vi "BMU诊断标定.vi"(8 "CAN端口":u16(ring), 9 "设备索引号":u16(ring), 10 "CAN卡类型":u32(ring)=21) -> ()   [LabVIEW 2013] (continued)
                              n3531 = control-ref of="项目信息"() -> (w5062:refnum<vi>)
                              n3532 = for {
                                N: w5055 -> [_]
                                tunnel: [""] -> w5061 mode=indexing
                              }
                              n3533 = Multiply(x=u8 1, y=w5056) -> (x*y=w5058:dbl)
                              n3534 = Add(x=w5058, y=u8 21) -> (x+y=w5054:dbl)
                              n3535 = call "表格数据输入-8.6.vi"("行数"=w5054, "列数"=u32 1, "字符串数组"=w5061, "表格引用"=w5062) -> ()  [unwired: 8 in]
                            }
                            frame "温度个数" {
                              n3536 = local read "从板个数"() -> (w5066:dbl)
                              n3537 = Increment(x=w5066) -> (x+1=w5065:dbl)
                              n3538 = control-ref of="项目信息"() -> (w5072:refnum<vi>)
                              n3539 = for {
                                N: w5065 -> [_]
                                tunnel: [""] -> w5071 mode=indexing
                              }
                              n3540 = Multiply(x=u8 2, y=w5066) -> (x*y=w5068:dbl)
                              n3541 = Add(x=w5068, y=u8 22) -> (x+y=w5064:dbl)
                              n3542 = call "表格数据输入-8.6.vi"("行数"=w5064, "列数"=u32 1, "字符串数组"=w5071, "表格引用"=w5072) -> ()  [unwired: 8 in]
                            }
                            frame "温度起始值" {
                              n3543 = local read "从板个数"() -> (w5076:dbl)
                              n3544 = Increment(x=w5076) -> (x+1=w5075:dbl)
                              n3545 = control-ref of="项目信息"() -> (w5082:refnum<vi>)
                              n3546 = for {
                                N: w5075 -> [_]
                                tunnel: [""] -> w5081 mode=indexing
                              }
                              n3547 = Multiply(x=u8 3, y=w5076) -> (x*y=w5078:dbl)
                              n3548 = Add(x=w5078, y=u8 23) -> (x+y=w5074:dbl)
                              n3549 = call "表格数据输入-8.6.vi"("行数"=w5074, "列数"=u32 1, "字符串数组"=w5081, "表格引用"=w5082) -> ()  [unwired: 8 in]
                            }
                            frame "保险位置" {
                              n3550 = local read "从板个数"() -> (w5086:dbl)
                              n3551 = control-ref of="项目信息"() -> (w5092:refnum<vi>)
                              n3552 = for {
                                N: 10 -> [_]
                                tunnel: [""] -> w5091 mode=indexing
                              }
                              n3553 = Multiply(x=u8 4, y=w5086) -> (x*y=w5088:dbl)
                              n3554 = Add(x=w5088, y=u8 24) -> (x+y=w5085:dbl)
                              n3555 = call "表格数据输入-8.6.vi"("行数"=w5085, "列数"=u32 1, "字符串数组"=w5091, "表格引用"=w5092) -> ()  [unwired: 8 in]
                            }
                            frame "电池额定实际容量" {
                              w5094 = 0.0 ("值")
                              n3556 = control-ref of="电池实际容量(A)"() -> (w5095:refnum<vi>)
                              n3557 = control-ref of="电池额定容量(A)"() -> (w5096:refnum<vi>)
                              n3558 = property class="DigNum (严格)"(reference=w5095, "Value"=w5094) -> ()  [unwired: 1 in, 2 out]
                              n3559 = property class="DigNum (严格)"(reference=w5096, "Value"=w5094) -> ()  [unwired: 1 in, 2 out]
                            }
                            frame "SOC" {
                              n3560 = control-ref of="SOC(%)"() -> (w5097:refnum<vi>)
                              n3561 = property class="DigNum (严格)"(reference=w5097, "Value"=0.0 ("值")) -> ()  [unwired: 1 in, 2 out]
                            }
                            frame "配置文件版本" {
                              n3562 = control-ref of="配置文件版本"() -> (w5099:refnum<vi>)
                              n3563 = property class="Str"(reference=w5099, "Value"="" ("值")) -> ()  [unwired: 1 in, 2 out]
                            }
                            frame "参数修改记录" {
                              n3564 = control-ref of="使用者"() -> (w5102:refnum<vi>)
                              n3565 = control-ref of="系统时钟"() -> (w5103:refnum<vi>)
                              n3566 = property class="DigNum (严格)"(reference=w5102, "Value"=0.0 ("值")) -> ()  [unwired: 1 in, 2 out]
                              n3567 = property class="Str"(reference=w5103, "Value"="" ("值")) -> ()  [unwired: 1 in, 2 out]
                            }
                            frame "校正时钟" {
                              n3568 = control-ref of="系统时钟"() -> (w5105:refnum<vi>)
                              n3569 = property class="Str"(reference=w5105, "Value"="" ("值")) -> ()  [unwired: 1 in, 2 out]
                            }
                            frame "车牌号" {
                              n3570 = control-ref of="车架(牌)号"() -> (w5107:refnum<vi>)
                              n3571 = property class="Str"(reference=w5107, "Value"="" ("值")) -> ()  [unwired: 1 in, 2 out]
                            }
                            frame "SOH" {
                              n3572 = control-ref of="SOH(%)"() -> (w5110:refnum<vi>)
                              n3573 = property class="DigNum (严格)"(reference=w5110, "Value"=0.0 ("值")) -> ()  [unwired: 1 in, 2 out]
                            }
                            frame "一级故障阀值" {
                              n3574 = local write "一级故障"(T10 {"总电压过高"=0.0, "整组电压不均衡"=0.0, "SOC过高"=0.0, "单体电压过高"=0.0, "总电压过低"=0.0, "温度过高"=0.0, "温度过低"=0.0, "单组电压不均衡"=0.0, "整组温度不均衡"=0.0, "单组温度不均衡"=0.0, "单体电压过低"=0.0, "充电电流过高"=0.0, "放电电流过高"=0.0, "SOC过低"=0.0, "内阻过大"=0.0, "极柱温度过高"=0.0, "SOH过低"=0.0} ("一级故障")) -> ()
                            }
                            frame "二级故障阀值" {
                              n3575 = local write "一级故障 2"(T10 {"总电压过高"=0.0, "整组电压不均衡"=0.0, "SOC过高"=0.0, "单体电压过高"=0.0, "总电压过低"=0.0, "温度过高"=0.0, "温度过低"=0.0, "单组电压不均衡"=0.0, "整组温度不均衡"=0.0, "单组温度不均衡"=0.0, "单体电压过低"=0.0, "充电电流过高"=0.0, "放电电流过高"=0.0, "SOC过低"=0.0, "内阻过大"=0.0, "极柱温度过高"=0.0, "SOH过低"=0.0} ("一级故障")) -> ()
                            }
                            frame "三级故障阀值" {
                              n3576 = local write "一级故障 3"(T10 {"总电压过高"=0.0, "整组电压不均衡"=0.0, "SOC过高"=0.0, "单体电压过高"=0.0, "总电压过低"=0.0, "温度过高"=0.0, "温度过低"=0.0, "单组电压不均衡"=0.0, "整组温度不均衡"=0.0, "单组温度不均衡"=0.0, "单体电压过低"=0.0, "充电电流过高"=0.0, "放电电流过高"=0.0, "SOC过低"=0.0, "内阻过大"=0.0, "极柱温度过高"=0.0, "SOH过低"=0.0} ("一级故障")) -> ()
                            }
                            frame "加热控制参数" {
                              n3577 = local write "加热控制参数"(T11 {"风机开启温度"=0.0, "风机关闭温度"=0.0, "加热开启温度"=0.0, "加热关闭温度"=0.0, "风机开启温差"=0.0, "风机关闭温差"=0.0, "加热关闭温差"=0.0} ("加热控制参数")) -> ()
                            }
                            frame "充电控制参数" {
                              n3578 = local write "一级故障 5"(T12 {"最大允许单体电压"=0.0, "最大允许总电压"=0.0, "最小允许单体电压"=0.0, "最大允许充电电流"=0.0, "最小允许充电电流"=0.0, "最大允许充电温度"=0.0, "最小允许充电温度"=0.0, "电流步长"=0.0} ("一级故障 5")) -> ()
                            }
                            frame "电池信息1" {
                              w5116 = ""
                              w5117 = 0.0 ("电池串联")
                              n3579 = local read "电池信息"() -> (w5119:T13)
                              n3580 = Bundle By Name(cluster=w5119, "电池串联"=w5117, "电池并联"=w5117, "电池包额定容量"=w5117, "电池包额定能量(kWh)"=w5117, "电池包额定总电压"=w5117, "实际容量"=w5117, "电池厂家"=w5116, "电池类型"=w5116, "电池生产日期"=w5116) -> (w5118:T13)
                              n3581 = local write "电池信息"(w5118) -> ()
                            }
                            frame "电池包组号" {
                              n3582 = local read "电池信息"() -> (w5122:T13)
                              n3583 = Bundle By Name(cluster=w5122, "电池包组号"="") -> (w5121:T13)
                              n3584 = local write "电池信息"(w5121) -> ()
                            }
                            frame "充放电安时" {
                              w5123 = 0.0 ("累计充电总安时")
                              n3585 = local read "电池信息"() -> (w5125:T13)
                              n3586 = Bundle By Name(cluster=w5125, "累计充电总安时"=w5123, "累计放电总安时"=w5123) -> (w5124:T13)
                              n3587 = local write "电池信息"(w5124) -> ()
                            }
                            frame "电池充放电次数" {
                              w5126 = 0.0 ("累计充电总安时")
                              n3588 = local read "电池信息"() -> (w5128:T13)
                              n3589 = Bundle By Name(cluster=w5128, "电池充满次数"=w5126, "电池放空次数"=w5126, "电池充电次数"=w5126) -> (w5127:T13)
                              n3590 = local write "电池信息"(w5127) -> ()
                            }
                          }
                        }
                        frame "从板" {
                          n3591 = case shown="\"加热控制参数\"" w5129 {
                            frame "假", Default {
                            }
                            frame "电压起始值" {
                              n3592 = control-ref of="项目信息 2"() -> (w5131:refnum<vi>)
                              n3593 = for {
                                N: 1 -> [_]
                                tunnel: [""] -> w5134 mode=indexing
                              }
                              n3594 = call "表格数据输入-8.6.vi"("行数"=u32 0, "列数"=u32 1, "字符串数组"=w5134, "表格引用"=w5131) -> ()  [unwired: 8 in]
                            }
                            frame "通道电压节数" {
                              n3595 = control-ref of="项目信息 2"() -> (w5136:refnum<vi>)
                              n3596 = for {
                                N: 5 -> [_]
                                tunnel: [""] -> w5140 mode=indexing
                              }
                              n3597 = call "表格数据输入-8.6.vi"("行数"=u32 22, "列数"=u32 1, "字符串数组"=w5140, "表格引用"=w5136) -> ()  [unwired: 8 in]
                            }
                            frame "保险位置" {
                              n3598 = control-ref of="项目信息 2"() -> (w5142:refnum<vi>)
                              n3599 = for {
                                N: 20 -> [_]
                                tunnel: [""] -> w5146 mode=indexing
                              }
                              n3600 = call "表格数据输入-8.6.vi"("行数"=u32 2, "列数"=u32 1, "字符串数组"=w5146, "表格引用"=w5142) -> ()  [unwired: 8 in]
                            }
                            frame "温度起始值" {
                              n3601 = control-ref of="项目信息 2"() -> (w5148:refnum<vi>)
                              n3602 = for {
                                N: 1 -> [_]
                                tunnel: [""] -> w5152 mode=indexing
                              }
                              n3603 = call "表格数据输入-8.6.vi"("行数"=u32 1, "列数"=u32 1, "字符串数组"=w5152, "表格引用"=w5148) -> ()  [unwired: 8 in]
                            }
                            frame "加热控制参数" {
                              n3604 = local write "加热控制参数"(T11 {"风机开启温度"=0.0, "风机关闭温度"=0.0, "加热开启温度"=0.0, "加热关闭温度"=0.0, "风机开启温差"=0.0, "风机关闭温差"=0.0, "加热关闭温差"=0.0} ("加热控制参数")) -> ()
                            }
                            frame "一级故障阀值" {
                              n3605 = local write "一级故障 6"(T15 {"电压过高"=0.0, "电压过低"=0.0, "温度过高"=0.0, "温度过低"=0.0, "电压不均衡(V)"=0.0, "温度不均衡"=0.0, "SOC过低"=0.0} ("一级故障 6")) -> ()
                            }
                            frame "二级故障阀值" {
                              n3606 = local write "一级故障 7"(T15 {"电压过高"=0.0, "电压过低"=0.0, "温度过高"=0.0, "温度过低"=0.0, "电压不均衡(V)"=0.0, "温度不均衡"=0.0, "SOC过低"=0.0} ("一级故障 7")) -> ()
                            }
                            frame "三级故障阀值" {
                              n3607 = local write "一级故障 8"(T15 {"电压过高"=0.0, "电压过低"=0.0, "温度过高"=0.0, "温度过低"=0.0, "电压不均衡(V)"=0.0, "温度不均衡"=0.0, "SOC过低"=0.0} ("一级故障 7")) -> ()
                            }
                            frame "均衡参数" {
                              n3608 = local write "均衡参数"(T17 {"充电结束电压(90%)"=0.0, "充电结束电压(91%)"=0.0, "充电结束电压(92%)"=0.0, "充电结束电压(93%)"=0.0, "充电结束电压(94%)"=0.0, "均衡计算-电压高阀值1级"=0.0, "均衡计算-电压高阀值2级"=0.0, "均衡计算-电压低阀值1级"=0.0, "均衡计算-电压低阀值2级"=0.0, "均衡计算-最低电压阀值"=0.0, "均衡停止-最低电压阀值"=0.0, "均衡计算-电压极差阀值"=0.0, "充电结束电压(95%)"=0.0, "充电结束电压(96%)"=0.0, "充电结束电压(97%)"=0.0, "充电结束电压(98%)"=0.0, "充电结束电压(99%)"=0.0, "充电结束电压(100%)"=0.0} ("均衡参数")) -> ()
                            }
                            frame "均衡阀值" {
                              w5159 = sgl 0.0 ("均衡计算-电压高阀值1级")
                              n3609 = local read "均衡参数"() -> (w5160:T17)
                              n3610 = Bundle By Name(cluster=w5160, "均衡计算-电压高阀值1级"=w5159, "均衡计算-电压高阀值2级"=w5159, "均衡计算-电压低阀值1级"=w5159, "均衡计算-电压低阀值2级"=w5159, "均衡计算-最低电压阀值"=w5159, "均衡停止-最低电压阀值"=w5159, "均衡计算-电压极差阀值"=w5159) -> (w5161:T17)
                              n3611 = local write "均衡参数"(w5161) -> ()
                            }
                            frame "充电结束电压" {
                              w5162 = sgl 0.0 ("均衡计算-电压高阀值1级")
                              n3612 = local read "均衡参数"() -> (w5163:T17)
                              n3613 = Bundle By Name(cluster=w5163, "充电结束电压(90%)"=w5162, "充电结束电压(91%)"=w5162, "充电结束电压(92%)"=w5162, "充电结束电压(93%)"=w5162, "充电结束电压(94%)"=w5162, "充电结束电压(95%)"=w5162, "充电结束电压(96%)"=w5162, "充电结束电压(97%)"=w5162, "充电结束电压(98%)"=w5162, "充电结束电压(99%)"=w5162, "充电结束电压(100%)"=w5162) -> (w5164:T17)
                              n3614 = local write "均衡参数"(w5164) -> ()
                            }
                          }
                        }
                      }
                    }
                    frame #1 {
                      w5165 = FALSE ("流控帧")
                      w5166 = TRUE ("流控帧 2")
                      n3615 = global write "EV05全局变量1.vi" "写入超时"(w5165) -> ()
                      n3616 = global write "EV05全局变量1.vi" "流控帧"(w5165) -> ()
                      n3617 = local write "写?"(w5165) -> ()
                      n3618 = call <vilib>:"Set Busy.vi"("disable click? (T)"=w5165) -> ()  [unwired: 3 in, 8 out]
                      n3619 = local write "消除"(w5166) -> ()
                      n3620 = local write "控制1"(w5166) -> ()
                      n3621 = global write "EV05全局变量1.vi" "流控帧 2"(w5166) -> ()
                    }
                    frame #2 {
                      n3622 = Wait Until Next ms Multiple(millisecond multiple=u32 150 ("毫秒倍数")) -> ()  [unwired: 1 out]
                    }
                    frame #3 {
                      n3623 = local read "设备索引号"() -> (w5173:u16)
                      n3624 = local read "CAN卡类型"() -> (w5174:u32)
                      n3625 = local read "CAN端口"() -> (w5172:u16)
                      n3626 = stacked-sequence {
                        tunnel: w5174 -> [_ w5182]
                        tunnel: w5173 -> [_ w5181]
                        tunnel: w5172 -> [_ w5180]
                        tunnel: w5171 -> [_ w5179]
                        tunnel: w5170 -> [_ w5178]
                        tunnel: w5169 -> [_ w5177]
                        tunnel: w5168 -> [_ w5176]
                        frame #0 {
                        }
                        frame #1 {
                          n3627 = call "多帧发送机制(EV05).vi"("can卡类型"=w5182, "设备索引号"=w5181, "CAN端口"=w5180, "命令"=w5178, "板号"=w5177, "命令序号"=w5179, "输入数据"=w5176) -> ("错误输出"=w5175:errorcluster)  [unwired: 1 in, 11 out]
                          n3628 = call <vilib>:"Clear Errors.vi"("error in (no error)"=w5175) -> ()  [unwired: 6 in, 1 out]
                        }
                      }
                      "命令序号" <- w5171
                    }
                    frame #4 {
                      n3629 = while {
                        tunnel: [w5187] -> w5184
                        tunnel: [w5186] -> w5183
                        i -> [w5190]
                        stop <- w5187 stop-if-true
                        n3630 = local read "强制终止读写标记"() -> (w5185:bool)
                        n3631 = global read "EV05全局变量1.vi" "写入超时"() -> (w5186:bool)
                        n3632 = Greater Or Equal?(x=w5190, y=30) -> (x >= y?=w5188:bool)
                        n3633 = Compound Arithmetic op=OR(w5185, w5186, w5188) -> (w5187:bool)
                        n3634 = Wait Until Next ms Multiple(millisecond multiple=u32 100 ("毫秒倍数")) -> ()  [unwired: 1 out]
                      }
                    }
                    frame #5 {
                      n3635 = call <vilib>:"Unset Busy.vi"() -> ()  [unwired: 11 in, 1 out]
                      n3636 = case shown="假" w5192 {
                        tunnel: w5193 -> [w5196 _]
                        frame False {
                          n3637 = control-ref of="结果"() -> (w5195:refnum<vi>)
                          n3638 = Concatenate Strings(w5196, "     读取失败" ("字符串")) -> (w5198:string)
                          n3639 = Build Array(w5198) -> (w5194:string[])
                          n3640 = call "表格编辑.vi"("新元素/子数组"=w5194, "活动单元格:单元格背景色"=u32 16740749, "MCListbox引用句柄"=w5195) -> ()  [unwired: 9 out]
                        }
                        frame True {
                        }
                      }
                    }
                    frame #6 {
                      n3641 = Increment(x=w5202) -> (x+1=w5201:i32)
                      n3642 = Equal?(x=w5203, y=w5201) -> (x = y?=w5200:bool)
                      n3643 = case shown="真" w5200 {
                        frame False {
                        }
                        frame True {
                          n3644 = control-ref of="结果"() -> (w5205:refnum<vi>)
                          n3645 = Concatenate Strings("读取完成" ("字符串")) -> (w5207:string)
                          n3646 = Build Array(w5207) -> (w5204:string[])
                          n3647 = call "表格编辑.vi"("新元素/子数组"=w5204, "活动单元格:单元格背景色"=u32 21937, "MCListbox引用句柄"=w5205) -> ()  [unwired: 9 out]
                        }
                      }
                    }
                  }
                }
              }
            }
          }
          n3648 = stacked-sequence {
            tunnel: w4857 -> [_]
            frame #0 {
              n3649 = call <vilib>:"Unset Busy.vi"() -> ()  [unwired: 11 in, 1 out]
              n3650 = local write "强制终止读写标记"(FALSE ("强制停止")) -> ()
            }
          }
        }
        frame "全部读取" {
          n3651 = stacked-sequence {
            seq-local: [w5213 _ _] -> [_ _ w5768]
            seq-local: [w5212 _ _] -> [_ _ w5767]
            tunnel: [_ w5404 _] -> w5210
            frame #0 {
              n3652 = local read "主从选择"() -> (w5213:enum32{"主板", "从板"})
              n3653 = local read "路径"() -> (w5214:path)
              n3654 = Empty String/Path?(string/path=w5214) -> (empty?=w5212:bool)
              n3655 = disable-structure shown="禁用" {
                disable-tunnel: w5214 -> [w5217 _]
                disable-tunnel: w5212 -> [w5216 _]
                disable-tunnel: w5213 -> [w5215 _]
                frame Disabled {
                  n3656 = case shown="假" w5216 {
                    tunnel: w5217 -> [w5221 _]
                    tunnel: w5215 -> [w5220 _]
                    frame False {
                      n3657 = control-ref of="结果"() -> (w5218:refnum<vi>)
                      n3658 = call-poly <vilib>:"Read From Spreadsheet File.vi"("file path (dialog if empty)"=w5221) -> ("all rows"=w5219:string[][])  [unwired: 3 in, 7 out]
                      n3659 = case shown="\"主板\", 默认" w5220 {
                        tunnel: w5219 -> [w5223 w5318]
                        tunnel: w5218 -> [w5222 w5317]
                        frame "主板", Default {
                          n3660 = stacked-sequence {
                            tunnel: w5223 -> [w5232 w5256 w5313]
                            tunnel: w5222 -> [w5229 _ w5284]
                            frame #0 {
                              n3661 = Index Array(array=w5232, index (col)=3 ("禁用的索引 (列)")) -> (element=w5246:string[])  [unwired: 1 in]
                              n3662 = Index Array(array=w5232, index (col)=1 ("禁用的索引 (列)")) -> (element=w5252:string[])  [unwired: 1 in]
                              n3663 = Delete From Array(array=w5246, length=4 ("长度"), index=0 ("索引")) -> (deleted portion=w5243:string[], array with subset deleted=w5237:string[])
                              n3664 = Delete From Array(array=w5252, length=1 ("长度"), index=0 ("索引")) -> (deleted portion=w5249:string[], array with subset deleted=w5226:string[])
                              n3665 = Build Array("正在读取主板配置文件...") -> (w5230:string[])
                              n3666 = Index Array(array=w5237) -> (element #1=w5236:string, element #2=w5235:string, element #3=w5234:string, element #4=w5233:string)  [unwired: 4 in]
                              n3667 = for {
                                tunnel: w5243 -> [w5255] mode=indexing
                                tunnel: [w5254] -> w5242 mode=indexing
                                n3668 = Fract/Exp String To Number(string=w5255) -> (number=w5254:dbl)  [unwired: 4 out]
                              }
                              n3669 = Index Array(array=w5249) -> (element=w5248:string)  [unwired: 1 in]
                              n3670 = global write "读配置文件全局.vi" "表格输入"(w5226) -> ()
                              n3671 = call "表格编辑.vi"("新元素/子数组"=w5230, "活动单元格:单元格背景色"=u32 6618880, "MCListbox引用句柄"=w5229) -> ()  [unwired: 9 out]
                              n3672 = Decimal String To Number(string=w5248) -> (number=w5227:i32)  [unwired: 1 in, 2 out]
                              n3673 = global read "读配置文件全局.vi" "项目信息"() -> (w5225:T27)
                              n3674 = Index Array(array=w5242) -> (element #1=w5241:dbl, element #2=w5240:dbl, element #3=w5239:dbl, element #4=w5238:dbl)  [unwired: 4 in]
                              n3675 = global write "读配置文件全局.vi" "从板个数"(w5227) -> ()
                              n3676 = Bundle(cluster=w5225, "电池额定容量"=w5241, "电池实际容量"=w5240, "车牌号"=w5236, "配置文件版本"=w5235, "SOH"=w5238, "SOC"=w5239, "产品编号"=w5234, "系统时钟"=w5233) -> (w5224:T27)  [unwired: 1 out]
                              n3677 = global write "读配置文件全局.vi" "项目信息"(w5224) -> ()
                            }
                            frame #1 {
                              n3678 = Index Array(array=w5256, index (col)=3 ("禁用的索引 (列)")) -> (element=w5274:string[])  [unwired: 1 in]
                              n3679 = Index Array(array=w5256, index (col)=5 ("禁用的索引 (列)")) -> (element=w5268:string[])  [unwired: 1 in]
                              n3680 = for {
                                tunnel: w5268 -> [w5281] mode=indexing
                                tunnel: [w5280] -> w5267 mode=indexing
                                n3681 = Fract/Exp String To Number(string=w5281) -> (number=w5280:dbl)  [unwired: 4 out]
                              }
                              n3682 = Delete From Array(array=w5274, length=17 ("长度"), index=8 ("索引")) -> (deleted portion=w5272:string[])  [unwired: 1 out]
                              n3683 = for {
                                tunnel: w5272 -> [w5283] mode=indexing
                                tunnel: [w5282] -> w5270 mode=indexing
                                n3684 = Fract/Exp String To Number(string=w5283) -> (number=w5282:dbl)  [unwired: 4 out]
                              }
                              n3685 = global write "读配置文件全局.vi" "二级故障"(w5267) -> ()
                              n3686 = global write "读配置文件全局.vi" "一级故障"(w5270) -> ()
                              n3687 = Index Array(array=w5256, index (col)=7 ("禁用的索引 (列)")) -> (element=w5265:string[])  [unwired: 1 in]
                              n3688 = Index Array(array=w5256, index (col)=9 ("禁用的索引 (列)")) -> (element=w5262:string[])  [unwired: 1 in]
                              n3689 = for {
                                tunnel: w5265 -> [w5279] mode=indexing
                                tunnel: [w5278] -> w5264 mode=indexing
                                n3690 = Fract/Exp String To Number(string=w5279) -> (number=w5278:dbl)  [unwired: 4 out]
                              }
                              n3691 = for {
                                tunnel: w5262 -> [w5277] mode=indexing
                                tunnel: [w5276] -> w5261 mode=indexing
                                n3692 = Fract/Exp String To Number(string=w5277) -> (number=w5276:dbl)  [unwired: 4 out]
                              }
                              n3693 = Delete From Array(array=w5261, length=6 ("长度"), index=0 ("索引")) -> (deleted portion=w5258:dbl[], array with subset deleted=w5257:dbl[])
                              n3694 = global write "读配置文件全局.vi" "三级故障"(w5264) -> ()
                              n3695 = global write "读配置文件全局.vi" "加热控制参数"(w5258) -> ()
                              n3696 = global write "读配置文件全局.vi" "充电控制参数"(w5257) -> ()
                            }
                            frame #2 {
                              n3697 = call <vilib>:"Unset Busy.vi"() -> ()  [unwired: 2 in, 10 out]
                              n3698 = Index Array(array=w5313, index (col)=11 ("禁用的索引 (列)")) -> (element=w5310:string[])  [unwired: 1 in]
                              n3699 = Delete From Array(array=w5310, length=6 ("长度"), index=0 ("索引")) -> (deleted portion=w5292:string[], array with subset deleted=w5291:string[])
                              n3700 = for {
                                tunnel: w5291 -> [w5316] mode=indexing
                                tunnel: [w5315] -> w5309 mode=indexing
                                n3701 = Fract/Exp String To Number(string=w5316) -> (number=w5315:dbl)  [unwired: 4 out]
                              }
                              n3702 = Index Array(array=w5292) -> (element #1=w5308:string, element #2=w5307:string, element #3=w5306:string, element #4=w5305:string, element #5=w5304:string, element #6=w5303:string)  [unwired: 6 in]
                              n3703 = Index Array(array=w5309) -> (element #1=w5302:dbl, element #2=w5301:dbl, element #3=w5300:dbl, element #4=w5299:dbl, element #5=w5298:dbl, element #6=w5297:dbl, element #7=w5296:dbl, element #8=w5295:dbl, element #9=w5294:dbl, element #10=w5293:dbl, element #11=w5288:dbl)  [unwired: 11 in]
                              n3704 = global read "读配置文件全局.vi" "电池信息"() -> (w5290:T28)
                              n3705 = Build Array("配置文件读取完成") -> (w5286:string[])
                              n3706 = Bundle(cluster=w5290, "电池串联"=w5302, "电池并联"=w5301, "累计放电总安时"=w5299, "电池包额定容量"=w5298, "电池包额定能量"=w5297, "电池包额定总电压"=w5296, "累计充电总安时"=w5300, "电池充满次数"=w5295, "电池放空次数"=w5294, "电池充电次数"=w5293, "电池生产日期"=w5308, "电池厂家"=w5307, "电池类型"=w5306, "电池包组号"=w5305, "电池包产权标识"=w5304, "电池应用车型"=w5303, "实际容量"=w5288) -> (w5289:T28)
                              n3707 = call "表格编辑.vi"("新元素/子数组"=w5286, "活动单元格:单元格背景色"=u32 6618880, "MCListbox引用句柄"=w5284) -> ()  [unwired: 9 out]
                              n3708 = global write "读配置文件全局.vi" "电池信息"(w5289) -> ()
                            }
                          }
                        }
                        frame "从板" {
                          n3709 = stacked-sequence {
                            tunnel: w5318 -> [w5326 w5354 w5398]
                            tunnel: w5317 -> [w5323 _ w5374]
                            frame #0 {
                              n3710 = Index Array(array=w5326, index (col)=1 ("禁用的索引 (列)")) -> (element=w5336:string[])  [unwired: 1 in]
                              n3711 = Index Array(array=w5326, index (col)=3 ("禁用的索引 (列)")) -> (element=w5330:string[])  [unwired: 1 in]
                              n3712 = Delete From Array(array=w5336, length=1 ("长度"), index=0 ("索引")) -> (deleted portion=w5333:string[], array with subset deleted=w5320:string[])
                              n3713 = Delete From Array(array=w5330, length=6 ("长度"), index=0 ("索引")) -> (deleted portion=w5327:string[])  [unwired: 1 out]
                              n3714 = for {
                                tunnel: w5327 -> [w5339] mode=indexing
                                tunnel: [w5338] -> w5319 mode=indexing
                                i -> [w5340]
                                n3715 = Fract/Exp String To Number(string=w5339, default (0 dbl)=w5340) -> (number=w5338:i32)  [unwired: 3 out]
                              }
                              n3716 = Index Array(array=w5333) -> (element=w5332:string)  [unwired: 1 in]
                              n3717 = global write "读配置文件全局2.vi" "表格"(w5320) -> ()
                              n3718 = Build Array("正在读取从板配置文件...") -> (w5324:string[])
                              n3719 = Decimal String To Number(string=w5332) -> (number=w5321:i32)  [unwired: 1 in, 2 out]
                              n3720 = call "表格编辑.vi"("新元素/子数组"=w5324, "活动单元格:单元格背景色"=u32 6618880, "MCListbox引用句柄"=w5323) -> ()  [unwired: 9 out]
                              n3721 = global write "读配置文件全局2.vi" "加热控制参数"(w5319) -> ()
                              n3722 = global write "读配置文件全局2.vi" "从板板号"(w5321) -> ()
                            }
                            frame #1 {
                              n3723 = Index Array(array=w5354, index (col)=3 ("禁用的索引 (列)")) -> (element=w5344:string[])  [unwired: 1 in]
                              n3724 = Array Subset(array=w5344, index=6 ("索引"), length=7 ("长度")) -> (w5351:string[])
                              n3725 = Array Subset(array=w5344, index=13 ("索引"), length=7 ("长度")) -> (w5350:string[])
                              n3726 = Array Subset(array=w5344, index=20 ("索引"), length=7 ("长度")) -> (w5345:string[])
                              n3727 = for {
                                tunnel: w5351 -> [w5361] mode=indexing
                                tunnel: [w5360] -> w5341 mode=indexing
                                n3728 = Fract/Exp String To Number(string=w5361) -> (number=w5360:dbl)  [unwired: 4 out]
                              }
                              n3729 = for {
                                tunnel: w5350 -> [w5359] mode=indexing
                                tunnel: [w5358] -> w5342 mode=indexing
                                n3730 = Fract/Exp String To Number(string=w5359) -> (number=w5358:dbl)  [unwired: 4 out]
                              }
                              n3731 = for {
                                tunnel: w5345 -> [w5357] mode=indexing
                                tunnel: [w5356] -> w5343 mode=indexing
                                n3732 = Fract/Exp String To Number(string=w5357) -> (number=w5356:dbl)  [unwired: 4 out]
                              }
                              n3733 = global write "读配置文件全局2.vi" "一级故障阀值"(w5341) -> ()
                              n3734 = global write "读配置文件全局2.vi" "二级故障阀值"(w5342) -> ()
                              n3735 = global write "读配置文件全局2.vi" "三级故障阀值"(w5343) -> ()
                            }
                            frame #2 {
                              n3736 = Index Array(array=w5398, index (col)=5 ("禁用的索引 (列)")) -> (element=w5396:string[])  [unwired: 1 in]
                              n3737 = Delete From Array(array=w5396, length=1 ("长度"), index=16 ("索引")) -> (deleted portion=w5392:string[], array with subset deleted=w5393:string[])
                              n3738 = for {
                                tunnel: w5393 -> [w5401] mode=indexing
                                tunnel: [w5400] -> w5397 mode=indexing
                                n3739 = Fract/Exp String To Number(string=w5401) -> (number=w5400:dbl)  [unwired: 4 out]
                              }
                              n3740 = Index Array(array=w5397) -> (element #1=w5391:dbl, element #2=w5390:dbl, element #3=w5389:dbl, element #4=w5388:dbl, element #5=w5387:dbl, element #6=w5386:dbl, element #7=w5385:dbl, element #8=w5384:dbl, element #9=w5383:dbl, element #10=w5382:dbl, element #11=w5381:dbl, element #12=w5372:dbl, element #13=w5380:dbl, element #14=w5379:dbl, element #15=w5378:dbl, element #16=w5377:dbl, element #17=w5370:dbl, element #18=w5369:dbl, element #19=w5368:dbl, element #20=w5367:dbl, element #21=w5366:dbl, element #22=w5365:dbl)  [unwired: 22 in]
                              n3741 = Build Array("配置文件读取完成") -> (w5375:string[])
                              n3742 = Index Array(array=w5392, index=22 ("索引")) -> (element=w5371:string)
                              n3743 = global read "读配置文件全局2.vi" "电池组信息"() -> (w5363:T29)
                              n3744 = call "表格编辑.vi"("新元素/子数组"=w5375, "活动单元格:单元格背景色"=u32 6618880, "MCListbox引用句柄"=w5374) -> ()  [unwired: 9 out]
                              n3745 = Bundle(cluster=w5363, "电池类型"=w5391, "电池厂家"=w5390, "电池地区"=w5389, "电池组序号"=w5388, "电池包串联数"=w5387, "电池包并联数"=w5386, "电池包安时数"=w5385, "电池包序号"=w5384, "充电次数"=w5383, "充满电时间"=w5382, "放空时间"=w5381, "车牌号"=w5371, "最大允许单体电压"=w5372, "最大允许总电压"=w5380, "最大允许温度"=w5379, "最小允许温度"=w5378, "最大允许充电电流"=w5377, "最小允许充电电流"=w5370, "最小允许单体电压"=w5369, "电流步长"=w5368, "SOC"=w5367, "充电总安时"=w5366, "放电总这时"=w5365) -> (w5362:T29)
                              n3746 = call <vilib>:"Unset Busy.vi"() -> ()  [unwired: 2 in, 10 out]
                              n3747 = global write "读配置文件全局2.vi" "电池组信息"(w5362) -> ()
                            }
                          }
                        }
                      }
                    }
                    frame True {
                    }
                  }
                }
                frame Enabled {
                }
              }
              n3748 = case shown="\"从板\"" w5213 {
                frame "主板", Default {
                  w5402 = FALSE
                  n3749 = global write "读配置文件全局.vi" "SOC判定"(w5402) -> ()
                  n3750 = global write "读配置文件全局.vi" "SOH判定"(w5402) -> ()
                  n3751 = global write "读配置文件全局.vi" "车牌号判定"(w5402) -> ()
                  n3752 = global write "读配置文件全局.vi" "电池信息1判定"(w5402) -> ()
                  n3753 = global write "读配置文件全局.vi" "保险位置判定"(w5402) -> ()
                  n3754 = global write "读配置文件全局.vi" "产品编号判定"(w5402) -> ()
                  n3755 = global write "读配置文件全局.vi" "充放电安时判定"(w5402) -> ()
                  n3756 = global write "读配置文件全局.vi" "从板个数判定"(w5402) -> ()
                  n3757 = global write "读配置文件全局.vi" "电池包组号判定"(w5402) -> ()
                  n3758 = global write "读配置文件全局.vi" "电压个数判定"(w5402) -> ()
                  n3759 = global write "读配置文件全局.vi" "电压起始值判定"(w5402) -> ()
                  n3760 = global write "读配置文件全局.vi" "二级故障判定"(w5402) -> ()
                  n3761 = global write "读配置文件全局.vi" "三级故障判定"(w5402) -> ()
                  n3762 = global write "读配置文件全局.vi" "通道电压数判定"(w5402) -> ()
                  n3763 = global write "读配置文件全局.vi" "温度个数判定"(w5402) -> ()
                  n3764 = global write "读配置文件全局.vi" "一级故障判定"(w5402) -> ()
                  n3765 = global write "读配置文件全局.vi" "温度起始值判定"(w5402) -> ()
                  n3766 = global write "读配置文件全局.vi" "充电控制参数判定"(w5402) -> ()
                  n3767 = global write "读配置文件全局.vi" "电池充放电次数判定"(w5402) -> ()
                  n3768 = global write "读配置文件全局.vi" "加热控制参数判定"(w5402) -> ()
                  n3769 = global write "读配置文件全局.vi" "配置文件版本判定"(w5402) -> ()
                  n3770 = global write "读配置文件全局.vi" "电池额定实际容量判定"(w5402) -> ()
                }
                frame "从板" {
                  w5403 = FALSE
                  n3771 = disable-structure shown="禁用" {
                    frame Disabled {
                      n3772 = global read "读配置文件全局2.vi" "充电次数时间判定"() -> ()  [unwired: 1 in]
                      n3773 = global read "读配置文件全局2.vi" "电池包信息1判定"() -> ()  [unwired: 1 in]
                      n3774 = global read "读配置文件全局2.vi" "电池包序号判定"() -> ()  [unwired: 1 in]
                      n3775 = global read "读配置文件全局2.vi" "充放电安时判定"() -> ()  [unwired: 1 in]
                      n3776 = global read "读配置文件全局2.vi" "车牌号判定"() -> ()  [unwired: 1 in]
                      n3777 = global read "读配置文件全局2.vi" "充电参数判定"() -> ()  [unwired: 1 in]
                      n3778 = global read "读配置文件全局2.vi" "保险位置判定"() -> ()  [unwired: 1 in]
                    }
                    frame Enabled {
                    }
                  }
                  n3779 = global write "读配置文件全局2.vi" "从板号判定"(w5403) -> ()
                  n3780 = global write "读配置文件全局2.vi" "通道电压判定"(w5403) -> ()
                  n3781 = global write "读配置文件全局2.vi" "保险位置判定"(w5403) -> ()
                  n3782 = global write "读配置文件全局2.vi" "二级故障判定"(w5403) -> ()
                  n3783 = global write "读配置文件全局2.vi" "三级故障判定"(w5403) -> ()
                  n3784 = global write "读配置文件全局2.vi" "一级故障判定"(w5403) -> ()
                  n3785 = global write "读配置文件全局2.vi" "电压起始值判定"(w5403) -> ()
                  n3786 = global write "读配置文件全局2.vi" "温度起始值判定"(w5403) -> ()
                }
              }
            }
            frame #1 {
              (unwired) "均衡参数"
              # "去掉加热控制信息 20140106"
              n3787 = local read "主从选择"() -> (w5407:enum32{"主板", "从板"})
              n3788 = case shown="\"主板\", 默认" w5407 {
                tunnel: [string[] ["项目信息", "一级故障阀值", "二级故障阀值", "三级故障阀值", "加热控制信息", "充电控制信息", "电池信息"] string[] ["从板信息", "一级故障阀值", "二级故障阀值", "三级故障阀值"]] -> w5406
                frame "主板", Default {
                }
                frame "从板" {
                }
              }
              n3789 = Array Size(array=w5406) -> (size(s)=w5405:i32)
              n3790 = for {
                tunnel: w5406 -> [w5423] mode=indexing
                tunnel: w5407 -> [w5411]
                tunnel: w5405 -> [w5415]
                tunnel: [w5410] -> w5404
                i -> [w5412]
                n3791 = case shown="\"主板\", 默认" w5411 {
                  tunnel: [w5719 w5747] -> w5417
                  tunnel: [w5718 w5748] -> w5418
                  tunnel: w5423 -> [w5715 w5744]
                  tunnel: [u8 0 ("板号") w5745] -> w5422
                  tunnel: [u8 0 ("板号") u8 0 ("板号")] -> w5421
                  tunnel: [w5714 w5743] -> w5419
                  frame "主板", Default {
                    n3792 = case shown="\"项目信息\"" w5715 {
                      tunnel: [_ u8[] [1, 2, 3, 4, 5, 6, 13, 8, 7, 9, 10, 11, 12] u8[] [1] u8[] [2] u8[] [3] u8[] [1] u8[] [2] u8[] [1, 2, 3] u8[] [1, 2, 3, 4]] -> w5719
                      tunnel: [_ u8 128 ("命令") u8 129 ("命令") u8 129 ("命令") u8 129 ("命令") u8 130 ("命令") u8 130 ("命令") u8 131 ("命令") u8 132 ("命令")] -> w5718
                      tunnel: [_ string[] ["产品编号", "电压个数", "通道电压数", "电压起始值", "温度个数", "温度起始值", "保险位置", "电池额定实际容量", "SOC", "配置文件版本", "参数修改记录", "车牌号", "SOH"] string[] ["一级故障阀值"] string[] ["二级故障阀值"] string[] ["三级故障阀值"] string[] ["加热控制参数"] string[] ["充电控制参数"] _ string[] ["电池信息1", "电池包组号", "充放电安时", "电池充放电次数"]] -> w5714
                      frame "假", Default {
                      }
                      frame "项目信息" {
                      }
                      frame "一级故障阀值" {
                      }
                      frame "二级故障阀值" {
                      }
                      frame "三级故障阀值" {
                      }
                      frame "加热控制信息" {
                      }
                      frame "充电控制信息" {
                      }
                      frame "历史信息" {
                      }
                      frame "电池信息" {
                      }
                    }
                  }
                  frame "从板" {
                    n3793 = case shown="\"从板信息\"" w5744 {
                      tunnel: [_ u8 0 ("命令") u8 2 ("命令") u8 2 ("命令") u8 2 ("命令") u8 3 ("命令") u8 6 ("命令")] -> w5748
                      tunnel: [_ u8[] [6, 1, 2, 3, 4, 5] u8[] [1] u8[] [2] u8[] [3] u8[] [1, 2, 3, 4, 5, 6, 7] u8[] [1, 2]] -> w5747
                      tunnel: [_ string[] ["从板号", "电压起始值", "通道电压节数", "保险位置", "温度起始值", "加热控制参数"] string[] ["一级故障阀值"] string[] ["二级故障阀值"] string[] ["三级故障阀值"] string[] ["电池包信息1", "电池包序号", "充放电安时", "充电次数时间", "SOC", "车牌号", "充电参数"] string[] ["均衡阀值", "充电结束电压"]] -> w5743
                      frame "假", Default {
                      }
                      frame "从板信息" {
                      }
                      frame "一级故障阀值" {
                      }
                      frame "二级故障阀值" {
                      }
                      frame "三级故障阀值" {
                      }
                      frame "快换参数" {
                      }
                      frame "均衡参数" {
                      }
                    }
                    n3794 = local read "从板号"() -> (w5745:u8)
                  }
                }
                n3795 = Increment(x=w5412) -> (x+1=w5414:i32)
                n3796 = Equal?(x=w5415, y=w5414) -> (x = y?=w5413:bool)
                n3797 = case shown="\"从板\"" w5411 {
                  tunnel: w5412 -> [w5685 w5699]
                  frame "主板", Default {
                    n3798 = case shown="0, 默认" w5685 {
                      tunnel: [T8."项目信息" ("主从板") T8."一级故障阀值" ("主从板") T8."二级故障阀值" ("主从板") T8."三级故障阀值" ("主从板") T8."控制参数" ("主从板") T8."电池信息" ("主从板")] -> w5684
                      frame 0, Default {
                        n3799 = local write "1"(TRUE ("1")) -> ()
                      }
                      frame 1 {
                        n3800 = local write "1 2"(TRUE ("1 2")) -> ()
                      }
                      frame 2 {
                        n3801 = local write "1 3"(TRUE ("1 3")) -> ()
                      }
                      frame 3 {
                        n3802 = local write "1 4"(TRUE ("1 4")) -> ()
                      }
                      frame 4, 5 {
                        n3803 = local write "1 5"(TRUE ("1 5")) -> ()
                      }
                      frame 6 {
                        n3804 = local write "1 11"(TRUE ("1 11")) -> ()
                      }
                    }
                    n3805 = local write "主板2"(w5684) -> ()
                  }
                  frame "从板" {
                    n3806 = case shown="4" w5699 {
                      tunnel: [T21."从板信息" ("等级 2") T21."从板信息" ("等级 2") T21."一级故障阀值" ("等级 2") T21."二级故障阀值" ("等级 2") T21."三级故障阀值" ("等级 2") T21."快换参数" ("等级 2") T14."均衡参数" ("等级 2")] -> w5698
                      frame 99, Default {
                        n3807 = local write "1 6"(TRUE ("1 6")) -> ()
                      }
                      frame 0 {
                        n3808 = local write "1 6"(TRUE ("1 6")) -> ()
                      }
                      frame 1 {
                        n3809 = local write "1 7"(TRUE ("1 7")) -> ()
                      }
                      frame 2 {
                        n3810 = local write "1 8"(TRUE ("1 8")) -> ()
                      }
                      frame 3 {
                        n3811 = local write "1 9"(TRUE ("1 9")) -> ()
                      }
                      frame 5 {
                        n3812 = local write "1 10"(TRUE ("1 10")) -> ()
                      }
                      frame 4 {
                        n3813 = local write "1 12"(TRUE ("1 10")) -> ()
                      }
                    }
                    n3814 = local write "等级 2"(w5698) -> ()
                  }
                }
                n3815 = Array Size(array=w5417) -> (size(s)=w5416:i32)
                n3816 = local write "命令"(w5418) -> ()
                n3817 = Build Array(w5421) -> (w5420:u8[])
                n3818 = while {
                  tunnel: w5418 -> [w5455]
                  tunnel: w5422 -> [w5454]
                  tunnel: w5420 -> [w5453]
                  tunnel: w5416 -> [w5449]
                  tunnel: w5413 -> [w5452]
                  tunnel: w5411 -> [w5446]
                  tunnel: [w5445] -> w5410
                  shift-right: [w5444] -> _
                  shift-left: w5419 -> [w5425]
                  shift-right: [w5435] -> _
                  shift-left: w5417 -> [w5424]
                  i -> [w5450]
                  stop <- w5445 stop-if-true
                  n3819 = local read "强制终止读写标记"() -> (w5441:bool)
                  n3820 = Array Size(array=w5425) -> (size(s)=w5443:i32)
                  n3821 = Increment(x=w5450) -> (x+1=w5451:i32)
                  n3822 = Greater Than 0?(x=w5443) -> (x > 0?=w5442:bool)
                  n3823 = Equal?(x=w5449, y=w5451) -> (x = y?=w5447:bool)
                  n3824 = Not(x=w5441) -> (.not. x?=w5440:bool)
                  n3825 = And(x=w5440, y=w5442) -> (x .and. y?=w5439:bool)
                  n3826 = Delete From Array(array=w5425, length=1 ("长度"), index=0 ("索引")) -> (deleted portion=w5431:string[], array with subset deleted=w5436:string[])
                  n3827 = Index Array(array=w5431, index=0 ("索引")) -> (element=w5429:string)
                  n3828 = Delete From Array(array=w5424, length=1 ("长度"), index=0 ("索引")) -> (deleted portion=w5427:u8[], array with subset deleted=w5432:u8[])
                  n3829 = Index Array(array=w5427, index=0 ("索引")) -> (element=w5426:u8)
                  n3830 = case shown="真" w5439 {
                    tunnel: w5455 -> [_ w5471]
                    tunnel: w5426 -> [_ w5470]
                    tunnel: w5454 -> [_ w5469]
                    tunnel: w5453 -> [_ w5468]
                    tunnel: w5429 -> [_ w5467]
                    tunnel: w5452 -> [_ w5466]
                    tunnel: w5447 -> [_ w5465]
                    tunnel: w5446 -> [_ w5464]
                    tunnel: [string[] [] w5460] -> w5444
                    tunnel: w5436 -> [_ w5463]
                    tunnel: [u8[] [] w5458] -> w5435
                    tunnel: w5432 -> [_ w5462]
                    tunnel: w5425 -> [_ w5461]
                    tunnel: w5424 -> [_ w5459]
                    frame False {
                    }
                    frame True {
                      n3831 = while {
                        tunnel: w5471 -> [w5487]
                        tunnel: w5470 -> [w5486]
                        tunnel: w5469 -> [w5485]
                        tunnel: w5468 -> [w5484]
                        tunnel: w5467 -> [w5482]
                        tunnel: w5466 -> [w5481]
                        tunnel: w5465 -> [w5480]
                        tunnel: w5464 -> [w5479]
                        tunnel: w5463 -> [w5475]
                        tunnel: w5462 -> [w5473]
                        tunnel: w5461 -> [w5476]
                        tunnel: [w5477] -> w5460
                        tunnel: w5459 -> [w5474]
                        tunnel: [w5472] -> w5458
                        i -> [w5478]
                        stop <- w5483 stop-if-true
                        n3832 = stacked-sequence {
                          seq-local: [_ _ _ _ w5634 _ _] -> [_ _ _ _ _ w5650 _]
                          tunnel: w5487 -> [_ _ _ w5626 _ _ _]
                          tunnel: w5486 -> [_ _ _ w5625 _ _ _]
                          tunnel: w5485 -> [_ _ _ w5624 _ _ _]
                          tunnel: w5484 -> [_ _ _ w5623 _ _ _]
                          tunnel: [_ _ _ _ w5635 _ _] -> w5483
                          tunnel: w5482 -> [w5489 _ _ _ _ w5649 _]
                          tunnel: w5481 -> [_ _ _ _ _ _ w5677]
                          tunnel: w5480 -> [_ _ _ _ _ _ w5675]
                          tunnel: w5479 -> [w5488 _ _ _ _ _ _]
                          tunnel: w5478 -> [_ _ _ _ _ _ _]
                          tunnel: [_ _ _ _ _ w5648 _] -> w5477
                          tunnel: w5476 -> [_ _ _ _ _ w5647 _]
                          tunnel: w5475 -> [_ _ _ _ _ w5646 _]
                          tunnel: w5474 -> [_ _ _ _ _ w5645 _]
                          tunnel: w5473 -> [_ _ _ _ _ w5644 _]
                          tunnel: [_ _ _ _ _ w5643 _] -> w5472
                          frame #0 {
                            n3833 = case shown="\"主板\", 默认" w5488 {
                              tunnel: w5489 -> [w5490 w5581]
                              frame "主板", Default {
                                n3834 = case shown="\"电池包组号\"" w5490 {
                                frame "假", Default {
                                }
                                frame "产品编号" {
                                n3835 = control-ref of="产品编号"() -> (w5492:refnum<vi>)
                                n3836 = property class="Str"(reference=w5492, "Value"="") -> ()  [unwired: 1 in, 2 out]
                                }
                                frame "电压个数" {
                                n3837 = local read "从板个数"() -> (w5493:dbl)
                                n3838 = control-ref of="项目信息"() -> (w5497:refnum<vi>)
                                n3839 = for {
                                N: w5493 -> [_]
                                tunnel: [""] -> w5496 mode=indexing
                                }
                                n3840 = call "表格数据输入-8.6.vi"("行数"=u32 0, "列数"=u32 1, "字符串数组"=w5496, "表格引用"=w5497) -> ()  [unwired: 8 in]
                                }
                                frame "通道电压数" {
                                n3841 = disable-structure shown="禁用" {
                                frame Disabled {
                                n3842 = control-ref of="项目信息"() -> (w5503:refnum<vi>)
                                n3843 = for {
                                N: 20 -> [_]
                                tunnel: [""] -> w5502 mode=indexing
                                }
                                n3844 = local read "从板个数"() -> (w5504:dbl)
                                n3845 = Increment(x=w5504) -> (x+1=w5500:dbl)
                                n3846 = call "表格数据输入-8.6.vi"("行数"=w5500, "列数"=u32 1, "字符串数组"=w5502, "表格引用"=w5503) -> ()  [unwired: 8 in]
                                }
                                frame Enabled {
                                }
                                }
                                }
                                frame "电压起始值" {
                                n3847 = disable-structure shown="禁用" {
                                frame Disabled {
                                n3848 = local read "从板个数"() -> (w5508:dbl)
                                n3849 = Increment(x=w5508) -> (x+1=w5507:dbl)
                                n3850 = control-ref of="项目信息"() -> (w5514:refnum<vi>)
                                n3851 = for {
                                N: w5507 -> [_]
                                tunnel: [""] -> w5513 mode=indexing
                                }
                                n3852 = Multiply(x=u8 1, y=w5508) -> (x*y=w5510:dbl)
                                n3853 = Add(x=w5510, y=u8 21) -> (x+y=w5506:dbl)
                                n3854 = call "表格数据输入-8.6.vi"("行数"=w5506, "列数"=u32 1, "字符串数组"=w5513, "表格引用"=w5514) -> ()  [unwired: 8 in]
                                }
                                frame Enabled {
                                }
                                }
                                }
                                frame "温度个数" {
                                n3855 = local read "从板个数"() -> (w5518:dbl)
                                n3856 = Increment(x=w5518) -> (x+1=w5517:dbl)
                                n3857 = control-ref of="项目信息"() -> (w5524:refnum<vi>)
                                n3858 = for {
                                N: w5517 -> [_]
                                tunnel: [""] -> w5523 mode=indexing
                                }
                                n3859 = Multiply(x=u8 2, y=w5518) -> (x*y=w5520:dbl)
                                n3860 = Add(x=w5520, y=u8 22) -> (x+y=w5516:dbl)
                                n3861 = call "表格数据输入-8.6.vi"("行数"=w5516, "列数"=u32 1, "字符串数组"=w5523, "表格引用"=w5524) -> ()  [unwired: 8 in]
                                }
                                frame "温度起始值" {
                                n3862 = disable-structure shown="禁用" {
                                frame Disabled {
                                n3863 = local read "从板个数"() -> (w5528:dbl)
                                n3864 = Increment(x=w5528) -> (x+1=w5527:dbl)
                                n3865 = control-ref of="项目信息"() -> (w5534:refnum<vi>)
                                n3866 = for {
                                N: w5527 -> [_]
                                tunnel: [""] -> w5533 mode=indexing
                                }
                                n3867 = Multiply(x=u8 3, y=w5528) -> (x*y=w5530:dbl)
                                n3868 = Add(x=w5530, y=u8 23) -> (x+y=w5526:dbl)
                                n3869 = call "表格数据输入-8.6.vi"("行数"=w5526, "列数"=u32 1, "字符串数组"=w5533, "表格引用"=w5534) -> ()  [unwired: 8 in]
                                }
                                frame Enabled {
                                }
                                }
                                }
                                frame "保险位置" {
                                n3870 = local read "从板个数"() -> (w5538:dbl)
                                n3871 = control-ref of="项目信息"() -> (w5544:refnum<vi>)
                                n3872 = for {
                                N: 10 -> [_]
                                tunnel: [""] -> w5543 mode=indexing
                                }
                                n3873 = Multiply(x=u8 4, y=w5538) -> (x*y=w5540:dbl)
                                n3874 = Add(x=w5540, y=u8 24) -> (x+y=w5537:dbl)
                                n3875 = call "表格数据输入-8.6.vi"("行数"=w5537, "列数"=u32 1, "字符串数组"=w5543, "表格引用"=w5544) -> ()  [unwired: 8 in]
                                }
                                frame "电池额定实际容量" {
                                w5546 = 0.0 ("值")
                                n3876 = control-ref of="电池实际容量(A)"() -> (w5547:refnum<vi>)
                                n3877 = control-ref of="电池额定容量(A)"() -> (w5548:refnum<vi>)
                                n3878 = property class="DigNum (严格)"(reference=w5547, "Value"=w5546) -> ()  [unwired: 1 in, 2 out]
                                n3879 = property class="DigNum (严格)"(reference=w5548, "Value"=w5546) -> ()  [unwired: 1 in, 2 out]
                                }
                                frame "SOC" {
                                n3880 = control-ref of="SOC(%)"() -> (w5549:refnum<vi>)
                                n3881 = property class="DigNum (严格)"(reference=w5549, "Value"=0.0 ("值")) -> ()  [unwired: 1 in, 2 out]
                                }
                                frame "配置文件版本" {
                                n3882 = control-ref of="配置文件版本"() -> (w5551:refnum<vi>)
                                n3883 = property class="Str"(reference=w5551, "Value"="" ("值")) -> ()  [unwired: 1 in, 2 out]
                                }
                                frame "参数修改记录" {
                                n3884 = control-ref of="使用者"() -> (w5554:refnum<vi>)
                                n3885 = control-ref of="系统时钟"() -> (w5555:refnum<vi>)
                                n3886 = property class="DigNum (严格)"(reference=w5554, "Value"=0.0 ("值")) -> ()  [unwired: 1 in, 2 out]
